vi "ddsPDSetPtConvert.vi"(7 "Pre 3.0 AOM driver version?":bool, 10 "Register":dbl=8.0 min=0.0 max=15.0 step=1.0 format="%#.1f", 11 "PD Set-Point (V)":dbl[](array[numeric])=[0.0] min=0.0 max=3.3 step=0.0008 format="%.3g") -> (3 "Characters for FPGA":string="L8000\r\n")   [LabVIEW 2013, in "DDS9954_v2013.lvlib"]
uses:
  DDS9954_v2013.lvlib
  dataToAscii_16bit.vi
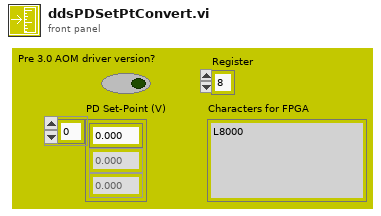
[diagram p1: front panel]
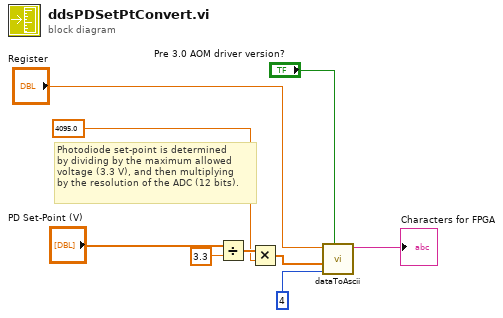
[diagram p0: block diagram]
diagram:
  # "Photodiode set-point is determined\nby dividing by the maximum allowed\nvoltage (3.3 V), and then multiplying\nby the resolution of the ADC (12 bits)."
  n1 = Divide(x="PD Set-Point (V)", y=3.3) -> (x/y=w8:dbl[])
  n2 = Multiply(x=w8, y=4095.0) -> (x*y=w3:dbl[])
  n3 = call-poly "dataToAscii.vi"("Pre 3.0 AOM driver version?"="Pre 3.0 AOM driver version?", "HEX min width (pre 3.0)"=u8 4, "Input Data"=w3, "Register"="Register") -> ("Characters to FPGA"=→"Characters for FPGA":string)  [unwired: 7 in]
